vi "Motion_Home Gantry.vi"(8 "error in":errorcluster, 10 "timeout (60s)":dbl[unit]=60.0 caption="Time Target (s)" format="%.1f", 11 "TCP address:port":string="192.168.0.3:502") -> (0 "error out":errorcluster, 2 "elapsed time":dbl[unit]=nan format="%.1f")   [LabVIEW 2010]
uses:
  Motion_Coils Typedef.ctl
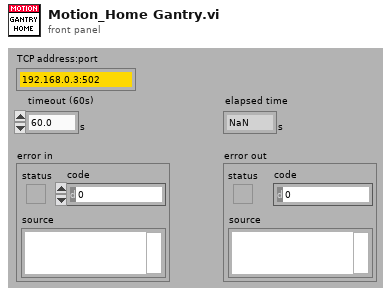
[diagram p1: front panel]
types:
  T1 = typedef "Motion_Coils Typedef.ctl" = u16
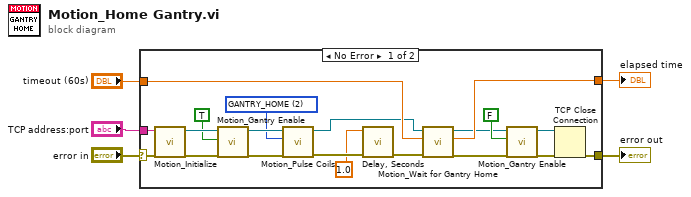
[diagram p0: block diagram]
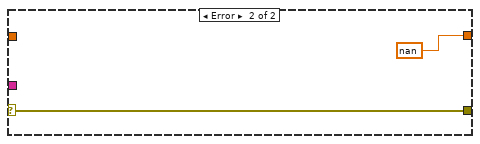
[diagram p2: hidden frame]
diagram:
  n1 = case shown="No Error" "error in" {
    selector: "error in" -> [w23 w27]
    tunnel: [w25 w27] -> w5
    tunnel: "TCP address:port" -> [w24 _]
    tunnel: [w13 dbl[unit] nan ("elapsed time")] -> w2
    tunnel: "timeout (60s)" -> [w10 _]
    frame No Error {
      w14 = T1 2 items=["GANTRY_ALARM_CLEAR", "GANTRY_ENABLE", "GANTRY_HOME", "GANTRY_GOTO", "LOADER_HOME", "LOADER_ALARM_CLEAR", "LOADER_ENABLE", "LOADER_GOTO_CONNECT", "LOADER_GOTO_LOAD", "LOADER_STOP"] ("Pulse Coil")
      n2 = call "Motion_Initialize.vi"("error in"=w23, "TCP address:port (192.168.0.3:502)"=w24) -> ("error out"=w22:errorcluster, "connection ID"=w21:refnum<k5>)  [unwired: 8 in]
      n3 = call "Motion_Gantry Enable.vi"("error in (no error)"=w22, "Enable? (T)"=TRUE, "TCP Connection Refnum in"=w21) -> ("error out"=w16:errorcluster, "TCP Connection Refnum (dup)"=w15:refnum<k5>)  [unwired: 7 in]
      n4 = call "Motion_Pulse Coils.vi"("error in"=w16, "Pulse Coil"=w14, "TCP refnum"=w15) -> ("error out"=w9:errorcluster, "TCP refnum dup"=w7:refnum<k5>)  [unwired: 7 in]
      n5 = call "Delay, Seconds.vi"("error in"=w9, "delay"=dbl[unit] 1.0) -> ("error out"=w8:errorcluster)  [unwired: 5 in, 1 out]
      n6 = call "Motion_Wait for Gantry Home.vi"("error in"=w8, "timeout (60s)"=w10, "TCP refnum"=w7) -> ("error out"=w12:errorcluster, "elapsed time"=w13:dbl[unit], "TCP refnum dup"=w11:refnum<k5>)  [unwired: 3 in, 3 out]
      n7 = call "Motion_Gantry Enable.vi"("error in (no error)"=w12, "Enable? (T)"=FALSE, "TCP Connection Refnum in"=w11) -> ("error out"=w17:errorcluster, "TCP Connection Refnum (dup)"=w18:refnum<k5>)  [unwired: 7 in]
      n8 = TCP Close Connection(connection ID=w18, error in (no error)=w17) -> (error out=w25:errorcluster)  [unwired: 1 in, 1 out]
    }
    frame Error {
    }
  }
  "error out" <- w5
  "elapsed time" <- w2
